vi "Open HTTP Client with API Key.vi"(8 "error in":errorcluster, 10 "API Key":string) -> (0 "error out":errorcluster, 3 "Refnum out":T1)   [LabVIEW 2023, in "LabVIEW AI Base.lvlib"]
uses:
  <vilib>/httpClient/ClientHandle.ctl
  LabVIEW AI Base.lvlib
  <vilib>/httpClient/LabVIEWHTTPClient.lvlib
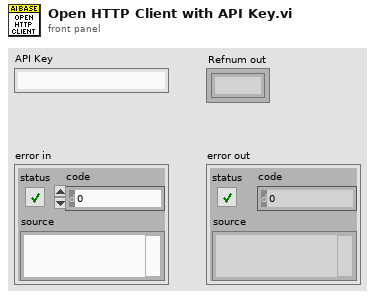
[diagram p1: front panel]
types:
  T1 = typedef "LabVIEWHTTPClient.lvlib/ClientHandle.ctl" = refnum<k1>
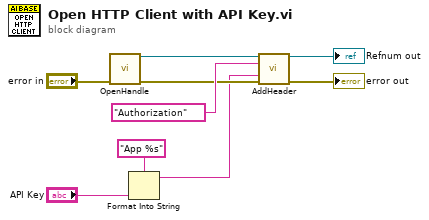
[diagram p0: block diagram]
diagram:
  n1 = call <vilib>:"OpenHandle.vi"("error in (no error)"="error in") -> ("client handle out"=w7:T1, "error out"=w5:errorcluster)  [unwired: 13 in]
  n2 = Format Into String(format string="App %s", "API Key") -> (resulting string=w3:string)  [unwired: 2 in, 1 out]
  n3 = call <vilib>:"AddHeader.vi"("client handle"=w7, "header"="Authorization", "value"=w3, "error in (no error)"=w5) -> ("client handle out"=→"Refnum out":T1, "error out"=→"error out":errorcluster)  [unwired: 10 in]
